vi "23_2b.vi"() -> ()   [LabVIEW 2020]
uses:
  <vilib>/Analysis/1siggen.llb/Ramp Pattern by Delta.vi
  <vilib>/Analysis/NI_AALBase.lvlib
panel:
  out "x-y":u32
  out "Count":i32
  in  "Cups":dbl=1000000.0 format="%#_13g"
  out "x*y":u64=54
  out "element 3":u64=9
  out "element 2":u64=6
  out "element":u64=1
  in  "Moves":i32=10000000
  in  "Switch":bool
  in  "Input":string="925176834"
  in  "Input Test":string="389125467"
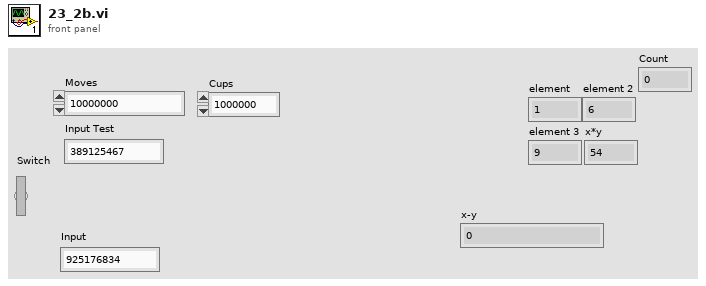
[diagram p1: front panel]
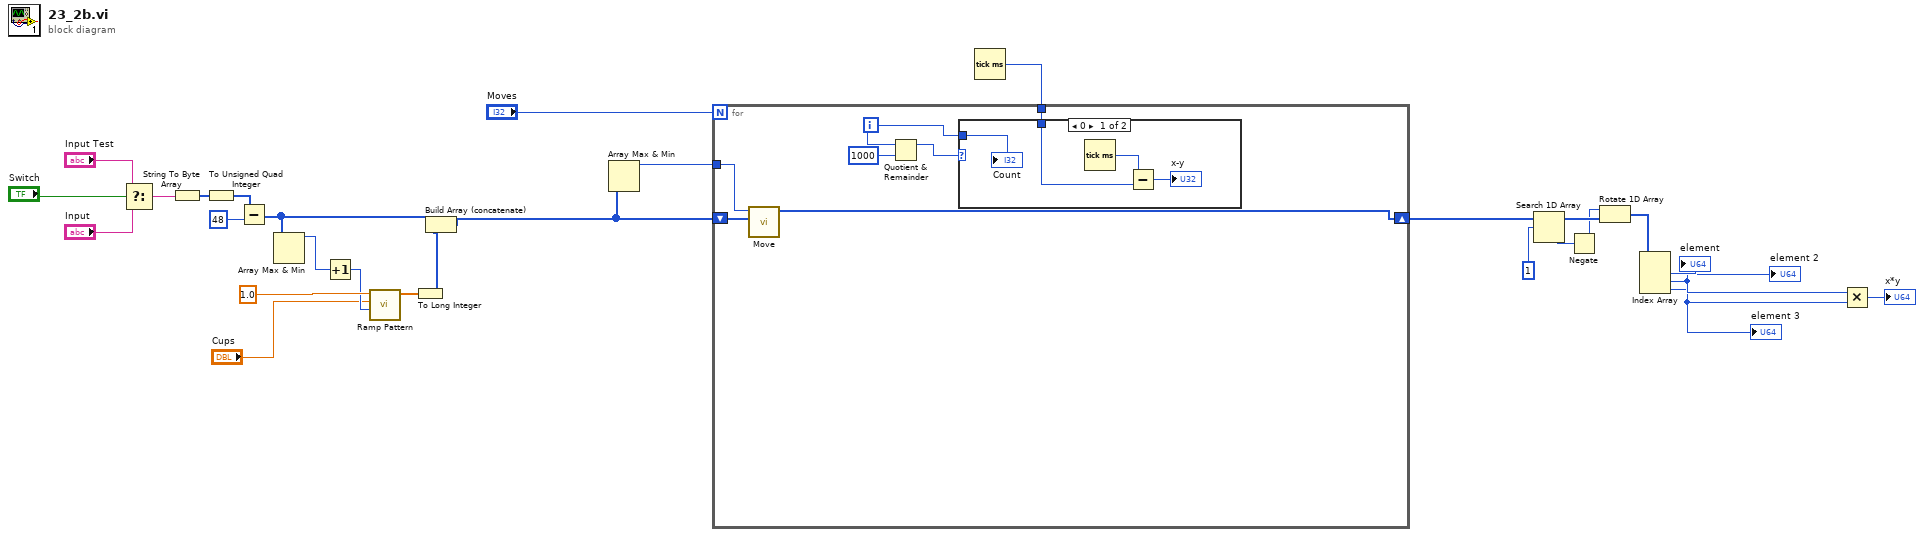
[diagram p0: block diagram]
diagram:
  n1 = Select(t="Input Test", s="Switch", f="Input") -> (s? t:f=w24:string)
  n2 = String To Byte Array(string=w24) -> (unsigned byte array=w23:u8[])
  n3 = To Unsigned Quad Integer(1:w23) -> (0:w15:u64[])
  n4 = Subtract(x=w15, y=u64 48) -> (x-y=w9:u64[])
  n5 = Array Max & Min(array=w9) -> (max value=w11:u64)  [unwired: 3 out]
  n6 = Increment(x=w11) -> (x+1=w12:u64)
  n7 = call-poly <vilib>:"Ramp Pattern.vi"("start"=w12, "end"="Cups", "delta"=1.0) -> ("Ramp Pattern"=w13:dbl[])  [unwired: 6 in, 2 out]
  n8 = To Long Integer(number=w13) -> (32bit integer=w8:i32[])
  n9 = Build Array (concatenate)(w9, w8) -> (w2:u64[])
  n10 = Array Max & Min(array=w2) -> (max value=w19:u64)  [unwired: 3 out]
  n11 = Tick Count (ms)() -> (millisecond timer value=w1:u32)
  n12 = for {
    N: "Moves" -> [_]
    shift-right: [w33] -> w18
    shift-left: w2 -> [w34]
    tunnel: w19 -> [w32]
    tunnel: w1 -> [w28]
    i -> [w29]
    n13 = call "Move.vi"("Array in"=w34, "Numeric"=w32) -> ("Array out"=w33:u64[])  [unwired: 9 in]
    n14 = Quotient & Remainder(x=w29, y=1000) -> (x-y*floor(x/y)=w30:i32)  [unwired: 1 out]
    n15 = case shown="0" w30 {
      tunnel: w29 -> [w38 _]
      tunnel: w28 -> [w36 _]
      frame 0 {
        n16 = Tick Count (ms)() -> (millisecond timer value=w37:u32)
        n17 = Subtract(x=w37, y=w36) -> (x-y=→"x-y":u32)
        "Count" <- w38
      }
      frame Default {
      }
    }
  }
  n18 = Search 1D Array(1D array=w18, element=u64 1) -> (index of element=w17:i32)  [unwired: 1 in]
  n19 = Negate(x=w17) -> (-x=w16:i32)
  n20 = Rotate 1D Array(1:w18, 2:w16) -> (0:w7:u64[])
  n21 = Index Array(array=w7) -> (element #1=→"element":u64, element #2=w5:u64, element #3=w4:u64)  [unwired: 3 in]
  "element 2" <- w5
  "element 3" <- w4
  n22 = Multiply(x=w5, y=w4) -> (x*y=→"x*y":u64)
